vi "Kill all MsgQ.vi"(8 "error in (no error)":errorcluster) -> (0 "error out":errorcluster)   [LabVIEW 2013, in "Main MsgQ.lvlib"]
doc: "Kills each message queue defined in the enumerated list."
uses:
  Main MsgQ.lvlib
  MsgQ Loops enum.ctl
  Common/Interloop MessageQ/Message que instance modes enum.ctl
  Common/Interloop MessageQ/Interloop MessageQ.lvlib
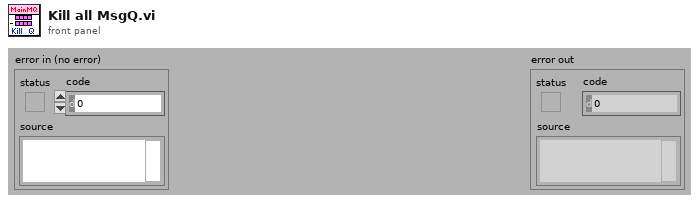
[diagram p1: front panel]
types:
  T1 = typedef "Main MsgQ.lvlib/MsgQ Loops enum.ctl" = enum16{"User Interface", "Image Acq"}
  T2 = typedef "Interloop MessageQ.lvlib/Message que instance modes enum.ctl" = enum16{"Initialize", "Broadcast Message", "Send Message", "Read Message", "Kill"}
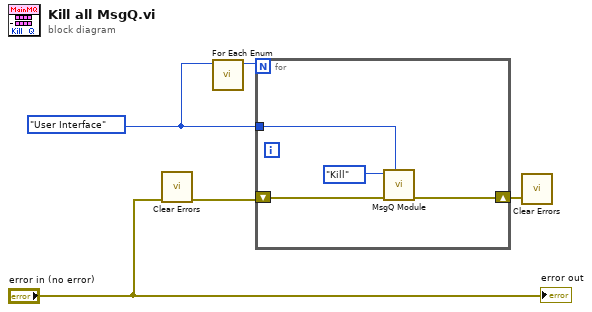
[diagram p0: block diagram]
diagram:
  w2 = MsgQ_Loops_enum."User Interface" ("MsgQ enum")
  n1 = call <vilib>:"Clear Errors.vi"("error in (no error)"="error in (no error)") -> ("error out"=w4:errorcluster)  [unwired: 6 out]
  n2 = call "For Each Enum.vi"("Enum In"=w2) -> ("# elements"=w5:i32)  [unwired: 10 out]
  n3 = for {
    N: w5 -> [_]
    shift-right: [w7] -> w1
    shift-left: w4 -> [w8]
    tunnel: w2 -> [w6]
    n4 = call "MsgQ Module.vi"("MsgQ enum"=w6, "error in (no error)"=w8, "Mode"=Message_que_instance_modes_enum."Kill") -> ("error out"=w7:errorcluster)  [unwired: 5 in, 3 out]
  }
  n5 = call <vilib>:"Clear Errors.vi"("error in (no error)"=w1) -> ()  [unwired: 6 in, 1 out]
  "error out" <- "error in (no error)"
